vi "MCLB_ItemIndex_Tests.vi"(11 "error in":errorcluster) -> (15 "error out":errorcluster)   [LabVIEW 2016, in "DronaTest.lvlib"]
uses:
  DronaTest.lvlib
  APIs/Stimulus/ControlValue/SetValueAuto.vi
  APIs/Stimulus/ControlValue/Controls/MC Listbox/SetValueByItemIndex.vi
  APIs/Assert/AssertControlValue/Equal.vi
  APIs/Get/GetControlRef/GetControlRefByPath.vi
  <vilib>/addons/_JKI Toolkits/Caraya/classes/Test/Test.lvclass
  Drona.lvlib
  <vilib>/SLL Toolkit/SLL Debug/SLL Debug.lvlib
  APIs/Assert/AssertControlValue/AssertControlValue.lvlib
  <vilib>/addons/_JKI Toolkits/Caraya/classes/Assert/Assert.lvclass
  APIs/Stimulus/ControlValue/Controls/MC Listbox/StimulusMCListbox.lvlib
  APIs/Get/GetControlRef/GetControlRef.lvlib
  APIs/Stimulus/ControlValue/ControlValue.lvlib
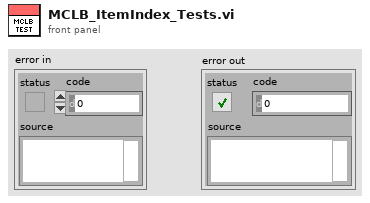
[diagram p1: front panel]
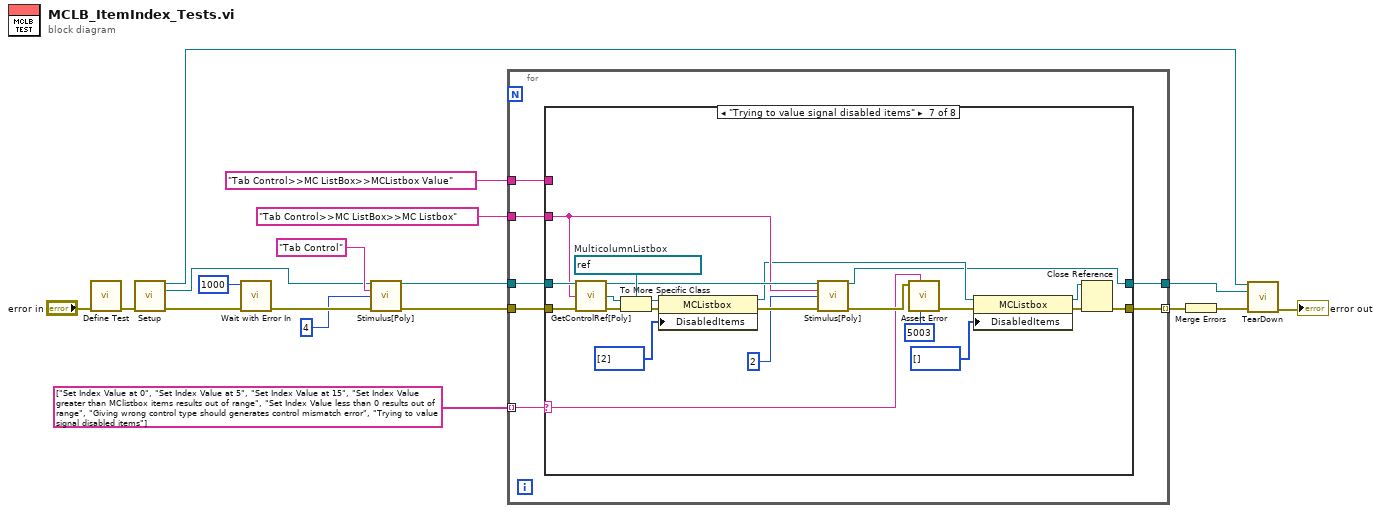
[diagram p0: block diagram]
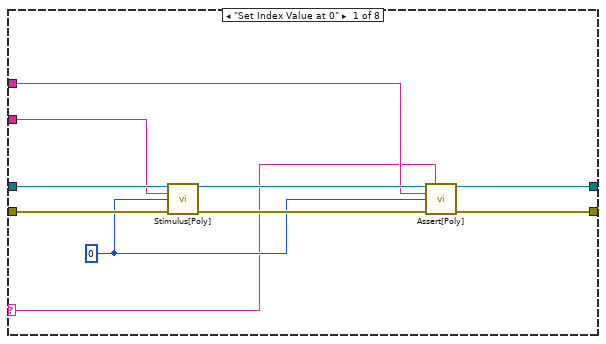
[diagram p2: hidden frame]
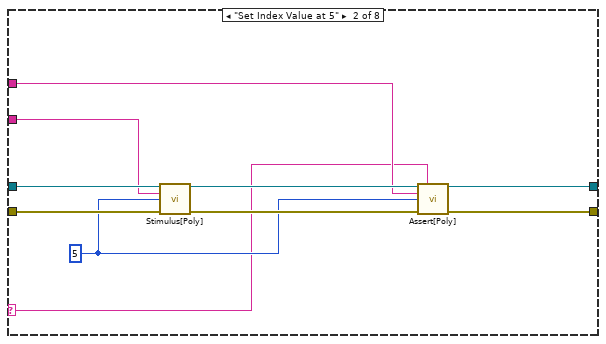
[diagram p3: hidden frame]
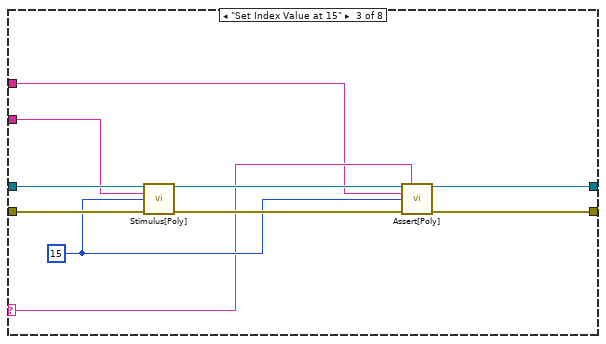
[diagram p4: hidden frame]
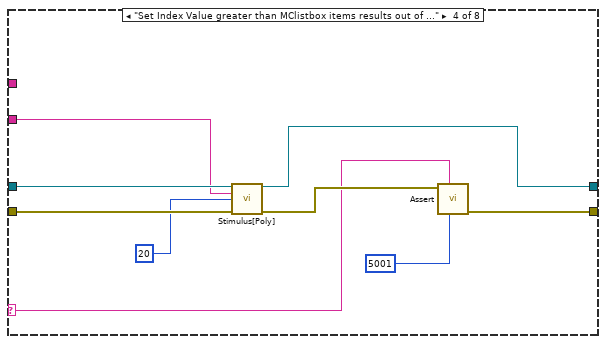
[diagram p5: hidden frame]
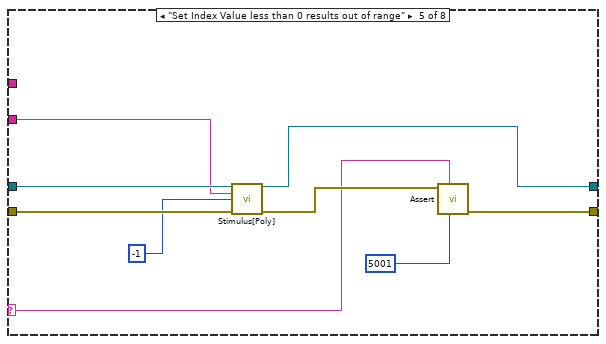
[diagram p6: hidden frame]
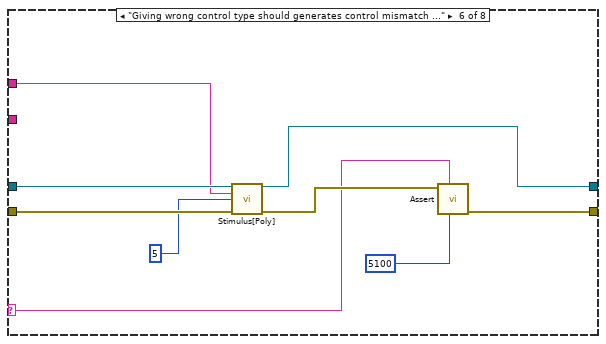
[diagram p7: hidden frame]
diagram:
  n1 = call <vilib>:"Define Test.vi"("error in (no error)"="error in") -> ("error out"=w7:errorcluster)  [unwired: 9 in, 1 out]
  n2 = call "Setup.vi"("error in (no error)"=w7) -> ("Application Ref"=w3:refnum<vi>, "VI out"=w5:refnum<vi>, "error out"=w6:errorcluster)  [unwired: 12 in]
  n3 = call <vilib>:"Wait with Error In.vi"("error in (no error)"=w6, "milliseconds to wait"=u32 1000) -> ("error out"=w16:errorcluster)  [unwired: 9 in]
  n4 = call-poly "Stimulus[Poly].vi"("VI Reference In"=w5, "Control Path"="Tab Control", "Value (Signaling)"=4, "error in"=w16) -> ("VI Reference Out"=w12:refnum<vi>, "error out"=w15:errorcluster)  [unwired: 10 in]
  n5 = for {
    tunnel: w12 -> [w24]
    tunnel: "Tab Control>>MC ListBox>>MC Listbox" ("Control Path") -> [w23]
    tunnel: "Tab Control>>MC ListBox>>MCListbox Value" ("Control Path") -> [w22]
    tunnel: string[] ["Set Index Value at 0", "Set Index Value at 5", "Set Index Value at 15", "Set Index Value greater than MClistbox items results out of range", "Set Index Value less than 0 results out of range", "Giving wrong control type should generates control mismatch error", "Trying to value signal disabled items"] -> [w20] mode=indexing
    tunnel: [w19] -> w2
    tunnel: w15 -> [w25]
    tunnel: [w21] -> w8 mode=indexing
    n6 = case shown="\"Trying to value signal disabled items\"" w20 {
      selector: w20 -> [w26 w36 w48 w58 w67 w77 w84 _]
      tunnel: w25 -> [w35 w45 w55 w64 w73 w82 w104 w106]
      tunnel: w24 -> [w34 w44 w54 w63 w72 w81 w103 w105]
      tunnel: w23 -> [w30 w40 w46 w61 w70 _ w94 _]
      tunnel: w22 -> [w29 w39 w47 _ _ w74 _ _]
      tunnel: [w28 w38 w50 w59 w68 w78 w89 w106] -> w21
      tunnel: [w27 w37 w49 w56 w65 w75 w87 w105] -> w19
      frame "Set Index Value at 0" {
        w31 = 0 ("Item Index")
        n7 = call-poly "Stimulus[Poly].vi"("VI Reference In"=w34, "Control Path"=w30, "Item Index"=w31, "Error In"=w35) -> ("VI Reference Out"=w32:refnum<vi>, "Error Out"=w33:errorcluster)  [unwired: 10 in]
        n8 = call-poly "Assert[Poly].vi"("VI Reference In"=w32, "Test Label"=w26, "Control Path"=w29, "Control Value"=w31, "Error In"=w33) -> ("VI Reference Out"=w27:refnum<vi>, "Error Out"=w28:errorcluster)  [unwired: 8 in, 1 out]
      }
      frame "Set Index Value at 5" {
        w41 = 5 ("Item Index")
        n9 = call-poly "Stimulus[Poly].vi"("VI Reference In"=w44, "Control Path"=w40, "Item Index"=w41, "Error In"=w45) -> ("VI Reference Out"=w42:refnum<vi>, "Error Out"=w43:errorcluster)  [unwired: 10 in]
        n10 = call-poly "Assert[Poly].vi"("VI Reference In"=w42, "Test Label"=w36, "Control Path"=w39, "Control Value"=w41, "Error In"=w43) -> ("VI Reference Out"=w37:refnum<vi>, "Error Out"=w38:errorcluster)  [unwired: 8 in, 1 out]
      }
      frame "Set Index Value at 15" {
        w51 = 15 ("Item Index")
        n11 = call-poly "Stimulus[Poly].vi"("VI Reference In"=w54, "Control Path"=w46, "Item Index"=w51, "Error In"=w55) -> ("VI Reference Out"=w52:refnum<vi>, "Error Out"=w53:errorcluster)  [unwired: 10 in]
        n12 = call-poly "Assert[Poly].vi"("VI Reference In"=w52, "Test Label"=w48, "Control Path"=w47, "Control Value"=w51, "Error In"=w53) -> ("VI Reference Out"=w49:refnum<vi>, "Error Out"=w50:errorcluster)  [unwired: 8 in, 1 out]
      }
      frame "Set Index Value greater than MClistbox items results out of range" {
        n13 = call-poly "Stimulus[Poly].vi"("VI Reference In"=w63, "Control Path"=w61, "Item Index"=20, "Error In"=w64) -> ("VI Reference Out"=w56:refnum<vi>, "Error Out"=w60:errorcluster)  [unwired: 10 in]
        n14 = call-poly <vilib>:"Assert.vi"("error code (1)"=5001, "Label"=w58, "Error?"=w60) -> ("error out"=w59:errorcluster)  [unwired: 7 in, 1 out]
      }
      frame "Set Index Value less than 0 results out of range" {
        n15 = call-poly "Stimulus[Poly].vi"("VI Reference In"=w72, "Control Path"=w70, "Item Index"=-1, "Error In"=w73) -> ("VI Reference Out"=w65:refnum<vi>, "Error Out"=w69:errorcluster)  [unwired: 10 in]
        n16 = call-poly <vilib>:"Assert.vi"("error code (1)"=5001, "Label"=w67, "Error?"=w69) -> ("error out"=w68:errorcluster)  [unwired: 7 in, 1 out]
      }
      frame "Giving wrong control type should generates control mismatch error" {
        n17 = call-poly "Stimulus[Poly].vi"("VI Reference In"=w81, "Control Path"=w74, "Item Index"=5, "Error In"=w82) -> ("VI Reference Out"=w75:refnum<vi>, "Error Out"=w79:errorcluster)  [unwired: 10 in]
        n18 = call-poly <vilib>:"Assert.vi"("error code (1)"=5100, "Label"=w77, "Error?"=w79) -> ("error out"=w78:errorcluster)  [unwired: 7 in, 1 out]
      }
      frame "Trying to value signal disabled items" {
        w99 = refnum<vi> refnum  # MulticolumnListbox
        n19 = call-poly "GetControlRef[Poly].vi"("VI Reference In"=w103, "Control Path"=w94, "error In"=w104) -> ("VI Reference Out"=w95:refnum<vi>, "Ctl Refnum"=w100:refnum<vi>, "error out"=w102:errorcluster)  [unwired: 10 in]
        n20 = To More Specific Class(target class=w99, reference=w100, error in=w102) -> (specific class reference=w98:refnum<vi>, error out=w101:errorcluster)
        n21 = property class="MCListbox"(reference=w98, error in=w101, "DisabledItems"=i32[] [2] ("Disabled Items")) -> (reference out=w91:refnum<vi>, error out=w96:errorcluster)
        n22 = call-poly "Stimulus[Poly].vi"("VI Reference In"=w95, "Control Path"=w94, "Item Index"=2, "Error In"=w96) -> ("VI Reference Out"=w87:refnum<vi>, "Error Out"=w86:errorcluster)  [unwired: 10 in]
        n23 = call <vilib>:"Assert Error.vi"("error code (1)"=5003, "Label"=w84, "Error?"=w86) -> ("error out"=w85:errorcluster)  [unwired: 7 in, 1 out]
        n24 = property class="MCListbox"(reference=w91, error in=w85, "DisabledItems"=i32[] [] ("Disabled Items")) -> (reference out=w88:refnum<vi>, error out=w92:errorcluster)
        n25 = Close Reference(reference=w88, error in (no error)=w92) -> (error out=w89:errorcluster)
      }
      frame Default {
      }
    }
  }
  n26 = Merge Errors(w8) -> (w4:errorcluster)
  n27 = call "TearDown.vi"("Application Ref"=w3, "VI in"=w2, "error in (no error)"=w4) -> ("error out"=→"error out":errorcluster)  [unwired: 12 in]
